vi "ma_Initial guess for tone estimation.vi"   [LabVIEW 2020, in "NI_MAPro.lvlib"]
uses:
  NI_MAPro.lvlib
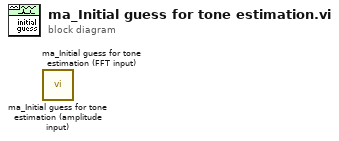
[diagram p0: block diagram]
diagram:
  n1 = call "ma_Initial guess for tone estimation (amplitude input).vi"() -> ()  [unwired: 2 in, 2 out]
  n2 = call "ma_Initial guess for tone estimation (FFT input).vi"() -> ()  [unwired: 2 in, 2 out]
